vi "FPGA_DMAWriteRate.vi"(8 "error in (no error)":errorcluster, 10 "Rate":u32, 11 "DMADevRef In":T1) -> (0 "error out":errorcluster, 3 "DMADevRef Out":T1)   [LabVIEW 2017]
uses:
  <vilib>/Rock Robotics/SystemInterfaces/DMA/FPGA_DMADevRef.ctl
  <vilib>/Rock Robotics/SystemInterfaces/System/FPGA_SystemFPGA Ref Global.vi
  <vilib>/Utility/error.llb/Error Cluster From Error Code.vi
  <vilib>/rvi/errors/niLvFpgaAdjustHostInterfaceError.vi
  <vilib>/rvi/interface/nirviReadWriteControl/nirviReadWriteControl.xnode
  <vilib>/Rock Robotics/SystemInterfaces/System/FPGA_SystemFRC FPGA Ref.ctl
  NiFpgaLv.dll
  <vilib>/rvi/interface/Simulation/niFpgaSimulationCallBeginRW.vi
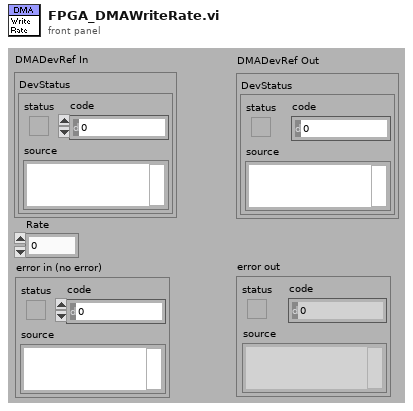
[diagram p1: front panel]
types:
  T1 = typedef "FPGA_DMADevRef.ctl" = cluster{"DevStatus":errorcluster}
  T2 = typedef "FPGA_SystemFRC FPGA Ref.ctl" = refnum<k20>
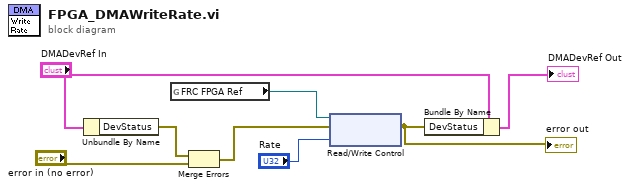
[diagram p0: block diagram]
diagram:
  n1 = Unbundle By Name("DMADevRef In") -> ("DevStatus"=w2:errorcluster)
  n2 = global read "FPGA_SystemFPGA Ref Global.vi" "FRC FPGA Ref"() -> (w4:T2)
  n3 = Merge Errors(w2, "error in (no error)") -> (w1:errorcluster)
  n4 = xnode "Read/Write Control"("FPGA VI Reference In"=w4, "error in"=w1, "DMA.Rate"="Rate") -> ("error out"=w6:errorcluster)  [unwired: 1 out]
  "error out" <- w6
  n5 = Bundle By Name(cluster="DMADevRef In", "DevStatus"=w6) -> (→"DMADevRef Out":T1)
